vi "greedyPath.vi"(8 "error in (no error)":errorcluster, 10 "ToVisit":T1[](array[typedef]), 11 "start":T1) -> (0 "error out":errorcluster, 2 "greedy Path":T1[](array[typedef]))   [LabVIEW 2014, in "Waypoint.lvclass"]
uses:
  <userlib>/AdvancedDataStructures/ClassBased/Applications/RouteSearch/Waypoint/Waypoint.lvclass
  <userlib>/AdvancedDataStructures/ClassBased/Applications/RouteSearch/Waypoint/point.ctl
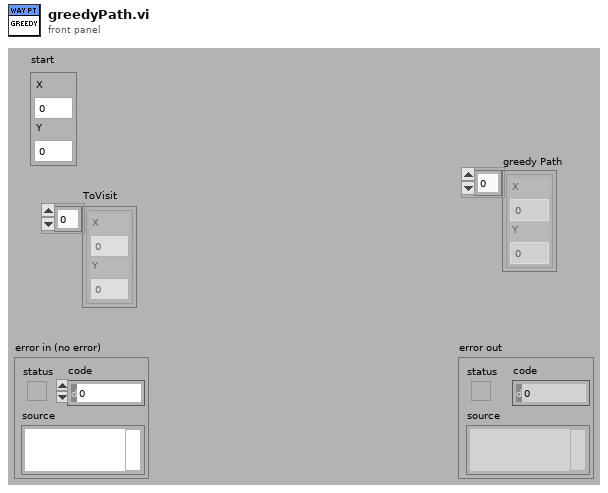
[diagram p1: front panel]
types:
  T1 = typedef "Waypoint.lvclass/point.ctl" = cluster{"X":dbl, "Y":dbl}
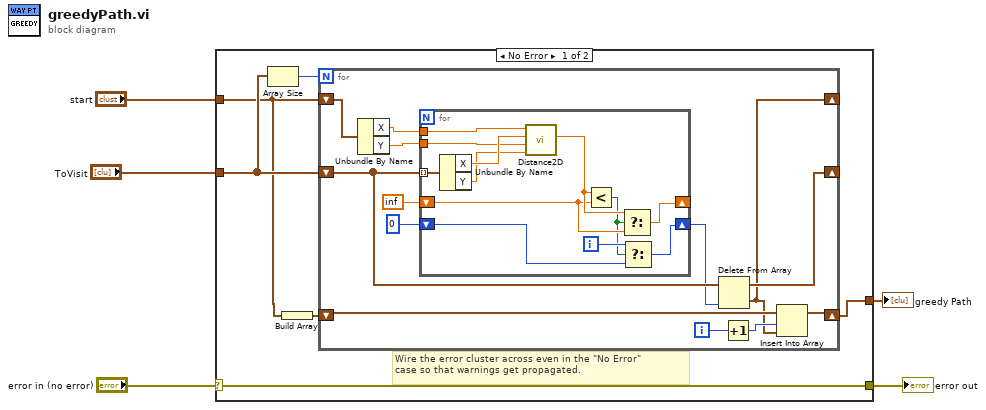
[diagram p0: block diagram]
diagram:
  n1 = case shown="No Error" "error in (no error)" {
    selector: "error in (no error)" -> [w11 w37]
    tunnel: [w11 w37] -> w4
    tunnel: "start" -> [w8 _]
    tunnel: "ToVisit" -> [w9 _]
    tunnel: [w6 _] -> w1
    frame No Error {
      # "Wire the error cluster across even in the \"No Error\"\ncase so that warnings get propagated."
      n2 = Array Size(array=w9) -> (size(s)=w10:i32)
      n3 = Build Array(w8) -> (w7:T1[])
      n4 = for {
        N: w10 -> [_]
        shift-right: [w14] -> _
        shift-left: w8 -> [w20]
        shift-right: [w17] -> _
        shift-left: w9 -> [w22]
        shift-right: [w13] -> w6
        shift-left: w7 -> [w16]
        i -> [w12]
        n5 = Unbundle By Name(w20) -> ("X"=w19:dbl, "Y"=w18:dbl)
        n6 = for {
          shift-right: [w29] -> _
          shift-left: inf -> [w30]
          tunnel: w19 -> [w35]
          tunnel: w18 -> [w33]
          tunnel: w22 -> [w36] mode=indexing
          shift-right: [w25] -> w21
          shift-left: 0 -> [w28]
          i -> [w27]
          n7 = Unbundle By Name(w36) -> ("X"=w34:dbl, "Y"=w32:dbl)
          n8 = call <userlib>:"Distance2D.vi"("y2"=w32, "y1"=w33, "x2"=w34, "x1"=w35) -> ("distance"=w31:dbl)  [unwired: 7 in]
          n9 = Less?(x=w31, y=w30) -> (x < y?=w26:bool)
          n10 = Select(t=w31, s=w26, f=w30) -> (s? t:f=w29:dbl)
          n11 = Select(t=w27, s=w26, f=w28) -> (s? t:f=w25:i32)
        }
        n12 = Delete From Array(array=w22, index=w21) -> (deleted portion=w14:T1, array with subset deleted=w17:T1[])  [unwired: 1 in]
        n13 = Increment(x=w12) -> (x+1=w15:i32)
        n14 = Insert Into Array(array=w16, index=w15, new element=w14) -> (w13:T1[])
      }
    }
    frame Error {
    }
  }
  "error out" <- w4
  "greedy Path" <- w1
